vi "S7_Init_TCP.vi"(8 "error in":errorcluster, 9 "Connection Timeout":u32=5000, 11 "IP Address":string) -> (0 "error out":errorcluster, 3 "TCP Connection Ref":refnum<k5>)   [LabVIEW 2018, in "S7 TCP.lvlib"]
uses:
  S7 TCP.lvlib
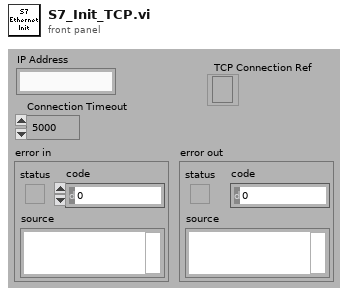
[diagram p1: front panel]
types:
  T1 = enum16{"Standard", "Buffered", "CRLF", "Immediate"}
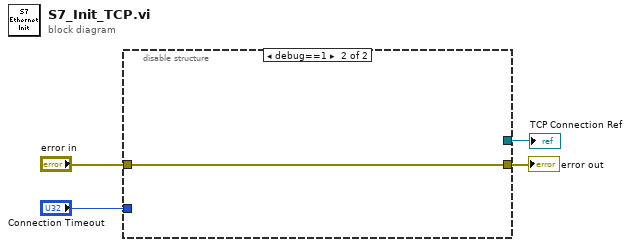
[diagram p0: block diagram]
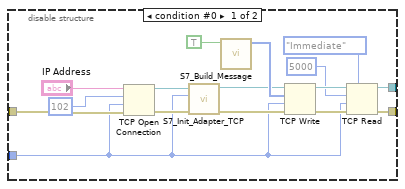
[diagram p2: hidden frame]
diagram:
  n1 = disable-structure shown="debug==1" {
    disable-tunnel: "error in" -> [w18 w21]
    disable-tunnel: [w9 _] -> w3
    disable-tunnel: [w8 w21] -> w2
    disable-tunnel: "Connection Timeout" -> [w6 _]
    frame condition #0 {
      n2 = TCP Open Connection(address="IP Address", remote port or service name=u16 102, timeout ms (60000)=w6, error in (no error)=w18) -> (connection ID=w17:refnum<k5>, error out=w16:errorcluster)  [unwired: 1 out]
      n3 = call "S7_Init_Adapter_TCP.vi"("error in"=w16, "Timeout"=w6, "TCP Connection Ref"=w17) -> ("error out"=w14:errorcluster, "TCP Connection Ref Out"=w13:refnum<k5>)  [unwired: 7 out]
      n4 = call "S7_Build_Message.vi"("Exchange PDU"=TRUE) -> ("S7 Ethernet Data"=w15:u8[])  [unwired: 2 in, 8 out]
      n5 = TCP Write(connection ID=w13, data in=w15, error in (no error)=w14, 9:w6) -> (connection ID out=w11:refnum<k5>, error out=w10:errorcluster)  [unwired: 1 out]
      n6 = TCP Read(connection ID=w11, bytes to read=5000, error in (no error)=w10, 7:T1."Immediate" ("mode (standard)"), 9:w6) -> (connection ID out=w9:refnum<k5>, error out=w8:errorcluster)  [unwired: 1 out]
    }
    frame condition #1 (active) {
    }
  }
  "error out" <- w2
  "TCP Connection Ref" <- w3
